vi "ConfigFlattenPositionsToXML.vi"(8 "error in":errorcluster, 11 "Position Array in":string[][](array[string])) -> (0 "error out":errorcluster, 3 "Position XML":string)   [LabVIEW 2018, in "Config.lvlib"]
uses:
  Config.lvlib
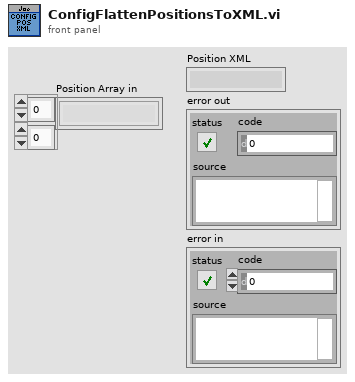
[diagram p1: front panel]
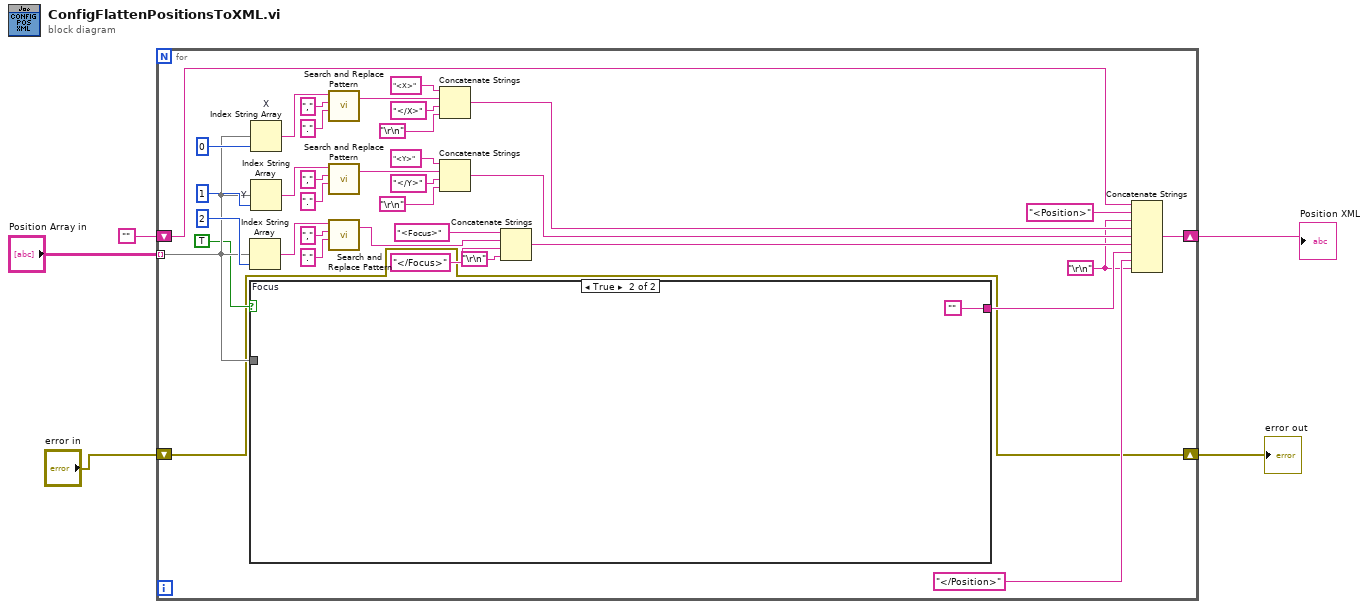
[diagram p0: block diagram]
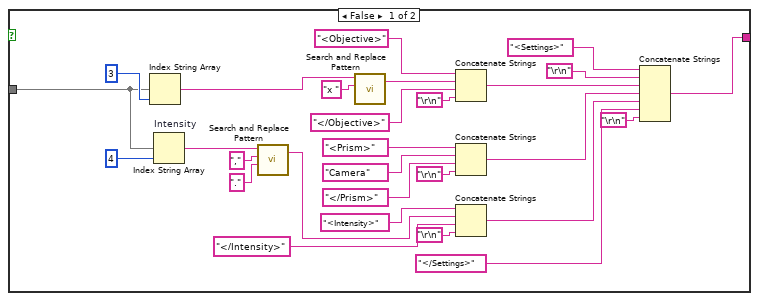
[diagram p2: hidden frame]
diagram:
  n1 = for {
    tunnel: "Position Array in" -> [w11] mode=indexing
    shift-right: [w33] -> w5
    shift-left: "" -> [w7]
    shift-right: [w6] -> w2
    shift-left: "error in" -> [w6]
    w8 = "\r\n"
    n2 = Index String Array "Focus"(1:2 ("index"), 2:w11) -> (0:w18:string)  [unwired: 1 in]
    n3 = case shown="True" TRUE {
      tunnel: [w65 ""] -> w36
      tunnel: w11 -> [w42 _]
      frame False {
        n4 = Index String Array(1:3 ("index"), 2:w42) -> (0:w49:string)  [unwired: 1 in]
        n5 = Index String Array "Intensity"(1:4 ("index"), 2:w42) -> (0:w44:string)  [unwired: 1 in]
        n6 = call <vilib>:"Search and Replace Pattern.vi"("string"=w44, "regular expression (\"\")"="," ("regular expression (\"\")"), "replace string (\"\")"="." ("replace string (\"\")")) -> ("result string"=w43:string)  [unwired: 2 in, 1 out]
        n7 = call <vilib>:"Search and Replace Pattern.vi"("string"=w49, "regular expression (\"\")"="x " ("replace string (\"\")")) -> ("result string"=w47:string)  [unwired: 3 in, 1 out]
        n8 = Concatenate Strings("<Objective>" ("string"), w47, "</Objective>" ("string"), "\r\n") -> (w59:string)
        n9 = Concatenate Strings("<Prism>" ("output string"), "Camera" ("output string"), "</Prism>" ("output string"), "\r\n") -> (w54:string)
        n10 = Concatenate Strings("<Intensity>" ("output string"), w43, "</Intensity>", "\r\n") -> (w50:string)
        n11 = Concatenate Strings("<Settings>" ("string"), "\r\n", w59, w54, w50, "</Settings>" ("string"), "\r\n") -> (w65:string)
      }
      frame True {
      }
    }
    n12 = Index String Array "X"(1:0 ("index"), 2:w11) -> (0:w21:string)  [unwired: 1 in]
    n13 = Index String Array "Y"(1:1 ("index"), 2:w11) -> (0:w27:string)  [unwired: 1 in]
    n14 = call <vilib>:"Search and Replace Pattern.vi"("string"=w21, "regular expression (\"\")"="," ("regular expression (\"\")"), "replace string (\"\")"="." ("replace string (\"\")")) -> ("result string"=w20:string)  [unwired: 2 in, 1 out]
    n15 = call <vilib>:"Search and Replace Pattern.vi"("string"=w27, "regular expression (\"\")"="," ("regular expression (\"\")"), "replace string (\"\")"="." ("replace string (\"\")")) -> ("result string"=w24:string)  [unwired: 2 in, 1 out]
    n16 = call <vilib>:"Search and Replace Pattern.vi"("string"=w18, "regular expression (\"\")"="," ("regular expression (\"\")"), "replace string (\"\")"="." ("replace string (\"\")")) -> ("result string"=w19:string)  [unwired: 2 in, 1 out]
    n17 = Concatenate Strings("<X>" ("string"), w20, "</X>" ("string"), "\r\n") -> (w35:string)
    n18 = Concatenate Strings("<Y>" ("string"), w24, "</Y>" ("string"), "\r\n") -> (w34:string)
    n19 = Concatenate Strings("<Focus>" ("string"), w19, "</Focus>" ("string"), "\r\n") -> (w10:string)
    n20 = Concatenate Strings(w7, "<Position>" ("string"), w8, w35, w34, w10, w36, "</Position>" ("string"), w8) -> (w33:string)
  }
  "Position XML" <- w5
  "error out" <- w2
